vi "Pre Launch Init.vi"(11 "DongWoo in":refnum<class "DongWoo.lvclass">) -> (0 "error out":errorcluster, 3 "DongWoo out":refnum<class "DongWoo.lvclass">)   [LabVIEW 2023, in "DongWoo_Spectrometer.lvlib" / "DongWoo.lvclass"]
doc: "(<B>Filename</B>: Actor Framework.lvlib:Actor.lvclass:Pre Launch Init.vi)\n\nDefines behavior that occurs after the Launch Nested Actor method is invoked but before the actor's Actor Core method begins running.\n\nBy default, this method does nothing. A descendant class may override it to define behavior."
uses:
  DongWoo.lvclass
  DongWoo.lvclass/DongWoo.ctl
  <vilib>/ActorFramework/Actor/Actor.lvclass
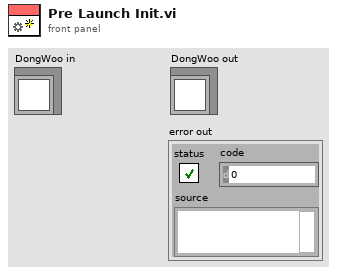
[diagram p1: front panel]
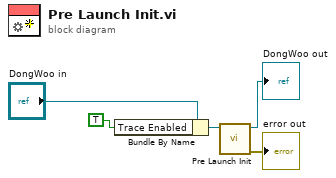
[diagram p0: block diagram]
diagram:
  n1 = Bundle By Name(cluster="DongWoo in", "Trace Enabled"=TRUE) -> (w1:refnum<class "DongWoo.lvclass">)
  n2 = call-parent "Pre Launch Init.vi"("Actor in"=w1) -> ("error out"=→"error out":errorcluster, "Actor out"=→"DongWoo out":refnum<class "DongWoo.lvclass">)  [unwired: 9 in]
